vi "complementary angle filter.vi"(1 "angular velocity":dbl format="%.2f", 2 "acceleration":dbl) -> (0 "filtered angle":dbl format="%.2f")   [LabVIEW 2013]
uses:
  <vilib>/addons/control/pid/pid.llb/PID Control Input Filter (DBL).vi
  <vilib>/addons/control/pid/NI_PID_pid.lvlib
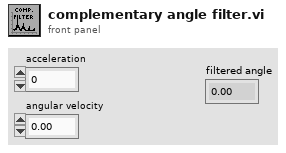
[diagram p1: front panel]
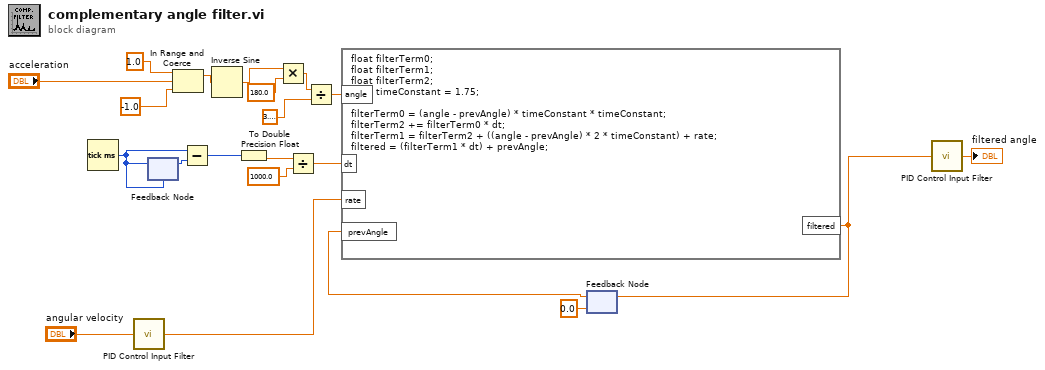
[diagram p0: block diagram]
diagram:
  n1 = Tick Count (ms)() -> (millisecond timer value=w12:u32)
  n2 = call-poly <vilib>:"PID Control Input Filter.vi"("input"="angular velocity") -> ("output"=w14:dbl)  [unwired: 4 in]
  n3 = feedback #1(w12) -> (w13:u32)
  n4 = feedback-in #1(w12) -> ()
  n5 = In Range and Coerce(upper limit=1.0, x="acceleration", lower limit=-1.0) -> (coerced(x)=w19:dbl)  [unwired: 1 out]
  n6 = Subtract(x=w12, y=w13) -> (x-y=w11:u32)
  n7 = Inverse Sine(1:w19) -> (0:w18:dbl)
  n8 = To Double Precision Float(number=w11) -> (double precision float=w7:dbl)
  n9 = Multiply(x=w18, y=180.0) -> (x*y=w17:dbl)
  n10 = Divide(x=w7, y=1000.0) -> (x/y=w5:dbl)
  n11 = Divide(x=w17, y=3.141592653589793) -> (x/y=w8:dbl)
  n12 = feedback #2(0.0 ("filtered")) -> (w9:dbl)
  n13 = formula code="float filterTerm0;\nfloat filterTerm1;\nfloat filterTerm2;\nfloat timeConstant = 1.75;\n\nfilterTerm0 = (angle - prevAngle) * timeConstant * timeConstant;\nfilterTerm2 += filterTerm0 * dt;\nfilterTerm1 = filterTerm2 + ((angle - prevAngle) * 2 * timeConstant) + rate;\nfiltered = (filterTerm1 * dt) + prevAngle;"("angle"=w8, "rate"=w14, "dt"=w5, "prevAngle"=w9) -> ("filtered"=w4:dbl)
  n14 = feedback-in #2(w4) -> ()
  n15 = call-poly <vilib>:"PID Control Input Filter.vi"("input"=w4) -> ("output"=→"filtered angle":dbl)  [unwired: 4 in]
